vi "Format CSV.vi"(8 "error in (no error)":errorcluster, 9 "delimiter":string=",", 10 "CSV File Input":path, 11 "Original CSV Format":enum16{"Format A", "Format B"}(ring)) -> (0 "error out":errorcluster, 1 "Parcel Length":i32[](array[numeric]), 2 "All Terminal Data":T1(array[cluster]))   [LabVIEW 2017] (continued)
"44:49.4", "44:49.5", "44:49.5", "44:49.5", "44:49.6", "44:49.6", "44:49.6", "44:49.7", "44:49.7", "44:49.7", "44:49.8", "44:49.8", "44:49.8", "44:49.9", "44:49.9", "44:49.9", "44:50.0", "44:50.0", "44:50.0", "44:50.1", "44:50.1", "44:50.1", "44:50.2", "44:50.2", "44:50.2", "44:50.3", "44:50.3", "44:50.3", "44:50.4", "44:50.4", "44:50.4", "44:50.5", "44:50.5", "44:50.5", "44:50.6", "44:50.6", "44:50.6", "44:50.7", "44:50.7", "44:50.7", "44:50.8", "44:50.8", "44:50.8", "44:50.9", "44:50.9", "44:50.9", "44:51.0", "44:51.0", "44:51.0", "44:51.1", "44:51.1", "44:51.1", "44:51.2", "44:51.2", "44:51.2", "44:51.3", "44:51.3", "44:51.3", "44:51.4", "44:51.4", "44:51.4", "44:51.5", "44:51.5", "44:51.5", "44:51.6", "44:51.6", "44:51.6", "44:51.7", "44:51.7", "44:51.7", "44:51.8", "44:51.8", "44:51.8", "44:51.9", "44:51.9", "44:51.9", "44:52.0", "44:52.0", "44:52.0", "44:52.1", "44:52.1", "44:52.1", "44:52.2", "44:52.2", "44:52.2", "44:52.3", "44:52.3", "44:52.3", "44:52.4", "44:52.4", "44:52.4", "44:52.5", "44:52.5", "44:52.5", "44:52.6", "44:52.6", "44:52.6", "44:52.7", "44:52.7", "44:52.7", "44:52.8", "44:52.8", "44:52.8", "44:52.9", "44:52.9", "44:52.9", "44:53.0", "44:53.0", "44:53.0", "44:53.1", "44:53.1", "44:53.1", "44:53.2", "44:53.2", "44:53.2", "44:53.3", "44:53.3", "44:53.3", "44:53.4", "44:53.4", "44:53.4", "44:53.5", "44:53.5", "44:53.5", "44:53.6", "44:53.6", "44:53.6", "44:53.7", "44:53.7", "44:53.7", "44:53.8", "44:53.8", "44:53.8", "44:53.9", "44:53.9", "44:53.9", "44:54.0", "44:54.0", "44:54.0", "44:54.1", "44:54.1", "44:54.1", "44:54.2", "44:54.2", "44:54.2", "44:54.3", "44:54.3", "44:54.3", "44:54.4", "44:54.4", "44:54.4", "44:54.5", "44:54.5", "44:54.5", "44:54.6", "44:54.6", "44:54.6", "44:54.7", "44:54.7", "44:54.7", "44:54.8", "44:54.8", "44:54.8", "44:54.9", "44:54.9", "44:54.9", "44:55.0", "44:55.0", "44:55.0", "44:55.1", "44:55.1", "44:55.1", "44:55.2", "44:55.2", "44:55.2", "44:55.3", "44:55.3", "44:55.3", "44:55.4", "44:55.4", "44:55.4", "44:55.5", "44:55.5", "44:55.5", "44:55.6", "44:55.6", "44:55.6", "44:55.7", "44:55.7", "44:55.7", "44:55.8", "44:55.8", "44:55.8", "44:55.9", "44:55.9", "44:55.9", "44:56.0", "44:56.0", "44:56.0", "44:56.1", "44:56.1", "44:56.1", "44:56.2", "44:56.2", "44:56.2", "44:56.3", "44:56.3", "44:56.3", "44:56.4", "44:56.4", "44:56.4", "44:56.5", "44:56.5", "44:56.5", "44:56.6", "44:56.6", "44:56.6", "44:56.7", "44:56.7", "44:56.7", "44:56.8", "44:56.8", "44:56.8", "44:56.9", "44:56.9", "44:56.9", "44:57.0", "44:57.0", "44:57.0", "44:57.1", "44:57.1", "44:57.1", "44:57.2", "44:57.2", "44:57.2", "44:57.3", "44:57.3", "44:57.3", "44:57.4", "44:57.4", "44:57.4", "44:57.5", "44:57.5", "44:57.5", "44:57.6", "44:57.6", "44:57.6", "44:57.7", "44:57.7", "44:57.7", "44:57.8", "44:57.8", "44:57.8", "44:57.9", "44:57.9", "44:57.9", "44:58.0", "44:58.0", "44:58.0", "44:58.1", "44:58.1", "44:58.1", "44:58.2", "44:58.2", "44:58.2", "44:58.3", "44:58.3", "44:58.3", "44:58.4", "44:58.4", "44:58.4", "44:58.5", "44:58.5", "44:58.5", "44:58.6", "44:58.6", "44:58.6", "44:58.7", "44:58.7", "44:58.7", "44:58.8", "44:58.8", "44:58.8", "44:58.9", "44:58.9", "44:58.9", "44:59.0", "44:59.0", "44:59.0", "44:59.1", "44:59.1", "44:59.1", "44:59.2", "44:59.2", "44:59.2", "44:59.3", "44:59.3", "44:59.3", "44:59.4", "44:59.4", "44:59.4", "44:59.5", "44:59.5", "44:59.5", "44:59.6", "44:59.6", "44:59.6", "44:59.7", "44:59.7", "44:59.7", "44:59.8", "44:59.8", "44:59.8", "44:59.9", "44:59.9", "44:59.9", "45:00.0", "45:00.0", "45:00.0", "45:00.1", "45:00.1", "45:00.1", "45:00.2", "45:00.2", "45:00.2", "45:00.3", "45:00.3", "45:00.3", "45:00.4", "45:00.4", "45:00.4", "45:00.5", "45:00.5", "45:00.5", "45:00.6", "45:00.6", "45:00.6", "45:00.7", "45:00.7", "45:00.7", "45:00.8", "45:00.8", "45:00.8", "45:00.9", "45:00.9", "45:00.9", "45:01.0", "45:01.0", "45:01.0", "45:01.1", "45:01.1", "45:01.1", "45:01.2", "45:01.2", "45:01.2", "45:01.3", "45:01.3", "45:01.3", "45:01.4", "45:01.4", "45:01.4", "45:01.5", "45:01.5", "45:01.5", "45:01.6", "45:01.6", "45:01.6", "45:01.7", "45:01.7", "45:01.7", "45:01.8", "45:01.8", "45:01.8", "45:01.9", "45:01.9", "45:01.9", "45:02.0", "45:02.0", "45:02.0", "45:02.1", "45:02.1", "45:02.1", "45:02.2", "45:02.2", "45:02.2", "45:02.3", "45:02.3", "45:02.3", "45:02.4", "45:02.4", "45:02.4", "45:02.5", "45:02.5", "45:02.5", "45:02.6", "45:02.6", "45:02.6", "45:02.7", "45:02.7", "45:02.7", "45:02.8", "45:02.8", "45:02.8", "45:02.9", "45:02.9", "45:02.9", "45:03.0", "45:03.0", "45:03.0", "45:03.1", "45:03.1", "45:03.1", "45:03.2", "45:03.2", "45:03.2", "45:03.3", "45:03.3", "45:03.3", "45:03.4", "45:03.4", "45:03.4", "45:03.5", "45:03.5", "45:03.5", "45:03.6", "45:03.6", "45:03.6", "45:03.7", "45:03.7", "45:03.7", "45:03.8", "45:03.8", "45:03.8", "45:03.9", "45:03.9", "45:03.9", "45:04.0", "45:04.0", "45:04.0", "45:04.1", "45:04.1", "45:04.1", "45:04.2", "45:04.2", "45:04.2", "45:04.3", "45:04.3", "45:04.3", "45:04.4", "45:04.4", "45:04.4", "45:04.5", "45:04.5", "45:04.5", "45:04.6", "45:04.6", "45:04.6", "45:04.7", "45:04.7", "45:04.7", "45:04.8", "45:04.8", "45:04.8", "45:04.9", "45:04.9", "45:04.9", "45:05.0", "45:05.0", "45:05.0", "45:05.1", "45:05.1", "45:05.1", "45:05.2", "45:05.2", "45:05.2", "45:05.3", "45:05.3", "45:05.3", "45:05.4", "45:05.4", "45:05.4", "45:05.5", "45:05.5", "45:05.5", "45:05.6", "45:05.6", "45:05.6", "45:05.7", "45:05.7", "45:05.7", "45:05.8", "45:05.8", "45:05.8", "45:05.9", "45:05.9", "45:05.9", "45:06.0", "45:06.0", "45:06.0", "45:06.1", "45:06.1", "45:06.1", "45:06.2", "45:06.2", "45:06.2", "45:06.3", "45:06.3", "45:06.3", "45:06.4", "45:06.4", "45:06.4", "45:06.5", "45:06.5", "45:06.5", "45:06.6", "45:06.6", "45:06.6", "45:06.7", "45:06.7", "45:06.7", "45:06.8", "45:06.8", "45:06.8", "45:06.9", "45:06.9", "45:06.9", "45:07.0", "45:07.0", "45:07.0", "45:07.1", "45:07.1", "45:07.1", "45:07.2", "45:07.2", "45:07.2", "45:07.3", "45:07.3", "45:07.3", "45:07.4", "45:07.4", "45:07.4", "45:07.5", "45:07.5", "45:07.5", "45:07.6", "45:07.6", "45:07.6", "45:07.7", "45:07.7", "45:07.7", "45:07.8", "45:07.8", "45:07.8", "45:07.9", "45:07.9", "45:07.9", "45:08.0", "45:08.0", "45:08.0", "45:08.1", "45:08.1", "45:08.1", "45:08.2", "45:08.2", "45:08.2", "45:08.3", "45:08.3", "45:08.3", "45:08.4", "45:08.4", "45:08.4", "45:08.5", "45:08.5", "45:08.5", "45:08.6", "45:08.6", "45:08.6", "45:08.7", "45:08.7", "45:08.7", "45:08.8", "45:08.8", "45:08.8", "45:08.9", "45:08.9", "45:08.9", "45:09.0", "45:09.0", "45:09.0", "45:09.1", "45:09.1", "45:09.1", "45:09.2", "45:09.2", "45:09.2", "45:09.3", "45:09.3", "45:09.3", "45:09.4", "45:09.4", "45:09.4", "45:09.5", "45:09.5", "45:09.5", "45:09.6", "45:09.6", "45:09.6", "45:09.7", "45:09.7", "45:09.7", "45:09.8", "45:09.8", "45:09.8", "45:09.9", "45:09.9", "45:09.9", "45:10.0", "45:10.0", "45:10.0", "45:10.1", "45:10.1", "45:10.1", "45:10.2", "45:10.2", "45:10.2", "45:10.3", "45:10.3", "45:10.3", "45:10.4", "45:10.4", "45:10.4", "45:10.5", "45:10.5", "45:10.5", "45:10.6", "45:10.6", "45:10.6", "45:10.7", "45:10.7", "45:10.7", "45:10.8", "45:10.8", "45:10.8", "45:10.9", "45:10.9", "45:10.9", "45:11.0", "45:11.0", "45:11.0", "45:11.1", "45:11.1", "45:11.1", "45:11.2", "45:11.2", "45:11.2", "45:11.3", "45:11.3", "45:11.3", "45:11.4", "45:11.4", "45:11.4", "45:11.5", "45:11.5", "45:11.5", "45:11.6", "45:11.6", "45:11.6", "45:11.7", "45:11.7", "45:11.7", "45:11.8", "45:11.8", "45:11.8", "45:11.9", "45:11.9", "45:11.9", "45:12.0", "45:12.0", "45:12.0", "45:12.1", "45:12.1", "45:12.1", "45:12.2", "45:12.2", "45:12.2", "45:12.3", "45:12.3", "45:12.3", "45:12.4", "45:12.4", "45:12.4", "45:12.5", "45:12.5", "45:12.5", "45:12.6", "45:12.6", "45:12.6", "45:12.7", "45:12.7", "45:12.7", "45:12.8", "45:12.8", "45:12.8", "45:12.9", "45:12.9", "45:12.9", "45:13.0", "45:13.0", "45:13.0", "45:13.1", "45:13.1", "45:13.1", "45:13.2", "45:13.2", "45:13.2", "45:13.3", "45:13.3", "45:13.3", "45:13.4", "45:13.4", "45:13.4", "45:13.5", "45:13.5", "45:13.5", "45:13.6", "45:13.6", "45:13.6", "45:13.7", "45:13.7", "45:13.7", "45:13.8", "45:13.8", "45:13.8", "45:13.9", "45:13.9", "45:13.9", "45:14.0", "45:14.0", "45:14.0", "45:14.1", "45:14.1", "45:14.1", "45:14.2", "45:14.2", "45:14.2", "45:14.3", "45:14.3", "45:14.3", "45:14.4", "45:14.4", "45:14.4", "45:14.5", "45:14.5", "45:14.5", "45:14.6", "45:14.6", "45:14.6", "45:14.7", "45:14.7", "45:14.7", "45:14.8", "45:14.8", "45:14.8", "45:14.9", "45:14.9", "45:14.9", "45:15.0", "45:15.0", "45:15.0", "45:15.1", "45:15.1", "45:15.1", "45:15.2", "45:15.2", "45:15.2", "45:15.3", "45:15.3", "45:15.3", "45:15.4", "45:15.4", "45:15.4", "45:15.5", "45:15.5", "45:15.5", "45:15.6", "45:15.6", "45:15.6", "45:15.7", "45:15.7", "45:15.7", "45:15.8", "45:15.8", "45:15.8", "45:15.9", "45:15.9", "45:15.9", "45:16.0", "45:16.0", "45:16.0", "45:16.1", "45:16.1", "45:16.1", "45:16.2", "45:16.2", "45:16.2", "45:16.3", "45:16.3", "45:16.3", "45:16.4", "45:16.4", "45:16.4", "45:16.5", "45:16.5", "45:16.5", "45:16.6", "45:16.6", "45:16.6", "45:16.7", "45:16.7", "45:16.7", "45:16.8", "45:16.8", "45:16.8", "45:16.9", "45:16.9", "45:16.9", "45:17.0", "45:17.0", "45:17.0", "45:17.1", "45:17.1", "45:17.1", "45:17.2", "45:17.2", "45:17.2", "45:17.3", "45:17.3", "45:17.3", "45:17.4", "45:17.4", "45:17.4", "45:17.5", "45:17.5", "45:17.5", "45:17.6", "45:17.6", "45:17.6", "45:17.7", "45:17.7", "45:17.7", "45:17.8", "45:17.8", "45:17.8", "45:17.9", "45:17.9", "45:17.9", "45:18.0", "45:18.0", "45:18.0", "45:18.1", "45:18.1", "45:18.1", "45:18.2", "45:18.2", "45:18.2", "45:18.3", "45:18.3", "45:18.3", "45:18.4", "45:18.4", "45:18.4", "45:18.5", "45:18.5", "45:18.5", "45:18.6", "45:18.6", "45:18.6", "45:18.7", "45:18.7", "45:18.7", "45:18.8", "45:18.8", "45:18.8", "45:18.9", "45:18.9", "45:18.9", "45:19.0", "45:19.0", "45:19.0", "45:19.1", "45:19.1", "45:19.1", "45:19.2", "45:19.2", "45:19.2", "45:19.3", "45:19.3", "45:19.3", "45:19.4", "45:19.4", "45:19.4", "45:19.5", "45:19.5", "45:19.5", "45:19.6", "45:19.6", "45:19.6", "45:19.7", "45:19.7", "45:19.7", "45:19.8", "45:19.8", "45:19.8", "45:19.9", "45:19.9", "45:19.9", "45:20.0", "45:20.0", "45:20.0", "45:20.1", "45:20.1", "45:20.1", "45:20.2", "45:20.2", "45:20.2", "45:20.3", "45:20.3", "45:20.3", "45:20.4", "45:20.4", "45:20.4", "45:20.5", "45:20.5", "45:20.5", "45:20.6", "45:20.6", "45:20.6", "45:20.7", "45:20.7", "45:20.7", "45:20.8", "45:20.8", "45:20.8", "45:20.9", "45:20.9", "45:20.9", "45:21.0", "45:21.0", "45:21.0", "45:21.1", "45:21.1", "45:21.1", "45:21.2", "45:21.2", "45:21.2", "45:21.3", "45:21.3", "45:21.3", "45:21.4", "45:21.4", "45:21.4", "45:21.5", "45:21.5", "45:21.5", "45:21.6", "45:21.6", "45:21.6", "45:21.7", "45:21.7", "45:21.7", "45:21.8", "45:21.8", "45:21.8", "45:21.9", "45:21.9", "45:21.9", "45:22.0", "45:22.0", "45:22.0", "45:22.1", "45:22.1", "45:22.1", "45:22.2", "45:22.2", "45:22.2", "45:22.3", "45:22.3", "45:22.3", "45:22.4", "45:22.4", "45:22.4", "45:22.5", "45:22.5", "45:22.5", "45:22.6", "45:22.6", "45:22.6", "45:22.7", "45:22.7", "45:22.7", "45:22.8", "45:22.8", "45:22.8", "45:22.9", "45:22.9", "45:22.9", "45:23.0", "45:23.0", "45:23.0", "45:23.1", "45:23.1", "45:23.1", "45:23.2", "45:23.2", "45:23.2", "45:23.3", "45:23.3", "45:23.3", "45:23.4", "45:23.4", "45:23.4", "45:23.5", "45:23.5", "45:23.5", "45:23.6", "45:23.6", "45:23.6", "45:23.7", "45:23.7", "45:23.7", "45:23.8", "45:23.8", "45:23.8", "45:23.9", "45:23.9", "45:23.9", "45:24.0", "45:24.0", "45:24.0", "45:24.1", "45:24.1", "45:24.1", "45:24.2", "45:24.2", "45:24.2", "45:24.3", "45:24.3", "45:24.3", "45:24.4", "45:24.4", "45:24.4", "45:24.5", "45:24.5", "45:24.5", "45:24.6", "45:24.6", "45:24.6", "45:24.7", "45:24.7", "45:24.7", "45:24.8", "45:24.8", "45:24.8", "45:24.9", "45:24.9", "45:24.9", "45:25.0", "45:25.0", "45:25.0", "45:25.1", "45:25.1", "45:25.1", "45:25.2", "45:25.2", "45:25.2", "45:25.3", "45:25.3", "45:25.3", "45:25.4", "45:25.4", "45:25.4", "45:25.5", "45:25.5", "45:25.5", "45:25.6", "45:25.6", "45:25.6", "45:25.7", "45:25.7", "45:25.7", "45:25.8", "45:25.8", "45:25.8", "45:25.9", "45:25.9", "45:25.9", "45:26.0", "45:26.0", "45:26.0", "45:26.1", "45:26.1", "45:26.1", "45:26.2", "45:26.2", "45:26.2", "45:26.3", "45:26.3", "45:26.3", "45:26.4", "45:26.4", "45:26.4", "45:26.5", "45:26.5", "45:26.5", "45:26.6", "45:26.6", "45:26.6", "45:26.7", "45:26.7", "45:26.7", "45:26.8", "45:26.8", "45:26.8", "45:26.9", "45:26.9", "45:26.9", "45:27.0", "45:27.0", "45:27.0", "45:27.1", "45:27.1", "45:27.1", "45:27.2", "45:27.2", "45:27.2", "45:27.3", "45:27.3", "45:27.3", "45:27.4", "45:27.4", "45:27.4", "45:27.5", "45:27.5", "45:27.5", "45:27.6", "45:27.6", "45:27.6", "45:27.7", "45:27.7", "45:27.7", "45:27.8", "45:27.8", "45:27.8", "45:27.9", "45:27.9", "45:27.9", "45:28.0", "45:28.0", "45:28.0", "45:28.1", "45:28.1", "45:28.1", "45:28.2", "45:28.2", "45:28.2", "45:28.3", "45:28.3", "45:28.3", "45:28.4", "45:28.4", "45:28.4", "45:28.5", "45:28.5", "45:28.5", "45:28.6", "45:28.6", "45:28.6", "45:28.7", "45:28.7", "45:28.7", "45:28.8", "45:28.8", "45:28.8", "45:28.9", "45:28.9", "45:28.9", "45:29.0", "45:29.0", "45:29.0", "45:29.1", "45:29.1", "45:29.1", "45:29.2", "45:29.2", "45:29.2", "45:29.3", "45:29.3", "45:29.3", "45:29.4", "45:29.4", "45:29.4", "45:29.5", "45:29.5", "45:29.5", "45:29.6", "45:29.6", "45:29.6", "45:29.7", "45:29.7", "45:29.7", "45:29.8", "45:29.8", "45:29.8", "45:29.9", "45:29.9", "45:29.9", "45:30.0", "45:30.0", "45:30.0", "45:30.1", "45:30.1", "45:30.1", "45:30.2", "45:30.2", "45:30.2", "45:30.3", "45:30.3", "45:30.3", "45:30.4", "45:30.4", "45:30.4", "45:30.5", "45:30.5", "45:30.5", "45:30.6", "45:30.6", "45:30.6", "45:30.7", "45:30.7", "45:30.7", "45:30.8", "45:30.8", "45:30.8", "45:30.9", "45:30.9", "45:30.9", "45:31.0", "45:31.0", "45:31.0", "45:31.1", "45:31.1", "45:31.1", "45:31.2", "45:31.2", "45:31.2", "45:31.3", "45:31.3", "45:31.3", "45:31.4", "45:31.4", "45:31.4", "45:31.5", "45:31.5", "45:31.5", "45:31.6", "45:31.6", "45:31.6", "45:31.7", "45:31.7", "45:31.7", "45:31.8", "45:31.8", "45:31.8", "45:31.9", "45:31.9", "45:31.9", "45:32.0", "45:32.0", "45:32.0", "45:32.1", "45:32.1", "45:32.1", "45:32.2", "45:32.2", "45:32.2", "45:32.3", "45:32.3", "45:32.3", "45:32.4", "45:32.4", "45:32.4", "45:32.5", "45:32.5", "45:32.5", "45:32.6", "45:32.6", "45:32.6", "45:32.7", "45:32.7", "45:32.7", "45:32.8", "45:32.8", "45:32.8", "45:32.9", "45:32.9", "45:32.9", "45:33.0", "45:33.0", "45:33.0", "45:33.1", "45:33.1", "45:33.1", "45:33.2", "45:33.2", "45:33.2", "45:33.3", "45:33.3", "45:33.3", "45:33.4", "45:33.4", "45:33.4", "45:33.5", "45:33.5", "45:33.5", "45:33.6", "45:33.6", "45:33.6", "45:33.7", "45:33.7", "45:33.7", "45:33.8", "45:33.8", "45:33.8", "45:33.9", "45:33.9", "45:33.9", "45:34.0", "45:34.0", "45:34.0", "45:34.1", "45:34.1", "45:34.1", "45:34.2", "45:34.2", "45:34.2", "45:34.3", "45:34.3", "45:34.3", "45:34.4", "45:34.4", "45:34.4", "45:34.5", "45:34.5", "45:34.5", "45:34.6", "45:34.6", "45:34.6", "45:34.7", "45:34.7", "45:34.7", "45:34.8", "45:34.8", "45:34.8", "45:34.9", "45:34.9", "45:34.9", "45:35.0", "45:35.0", "45:35.0", "45:35.1", "45:35.1", "45:35.1", "45:35.2", "45:35.2", "45:35.2", "45:35.3", "45:35.3", "45:35.3", "45:35.4", "45:35.4", "45:35.4", "45:35.5", "45:35.5", "45:35.5", "45:35.6", "45:35.6", "45:35.6", "45:35.7", "45:35.7", "45:35.7", "45:35.8", "45:35.8", "45:35.8", "45:35.9", "45:35.9", "45:35.9", "45:36.0", "45:36.0", "45:36.0", "45:36.1", "45:36.1", "45:36.1", "45:36.2", "45:36.2", "45:36.2", "45:36.3", "45:36.3", "45:36.3", "45:36.4", "45:36.4", "45:36.4", "45:36.5", "45:36.5", "45:36.5", "45:36.6", "45:36.6", "45:36.6", "45:36.7", "45:36.7", "45:36.7", "45:36.8", "45:36.8", "45:36.8", "45:36.9", "45:36.9", "45:36.9", "45:37.0", "45:37.0", "45:37.0", "45:37.1", "45:37.1", "45:37.1", "45:37.2", "45:37.2", "45:37.2", "45:37.3", "45:37.3", "45:37.3", "45:37.4", "45:37.4", "45:37.4", "45:37.5", "45:37.5", "45:37.5", "45:37.6", "45:37.6", "45:37.6", "45:37.7", "45:37.7", "45:37.7", "45:37.8", "45:37.8", "45:37.8", "45:37.9", "45:37.9", "45:37.9", "45:38.0", "45:38.0", "45:38.0", "45:38.1", "45:38.1", "45:38.1", "45:38.2", "45:38.2", "45:38.2", "45:38.3", "45:38.3", "45:38.3", "45:38.4", "45:38.4", "45:38.4", "45:38.5", "45:38.5", "45:38.5", "45:38.6", "45:38.6", "45:38.6", "45:38.7", "45:38.7", "45:38.7", "45:38.8", "45:38.8", "45:38.8", "45:38.9", "45:38.9", "45:38.9", "45:39.0", "45:39.0", "45:39.0", "45:39.1", "45:39.1", "45:39.1", "45:39.2", "45:39.2", "45:39.2", "45:39.3", "45:39.3", "45:39.3", "45:39.4", "45:39.4", "45:39.4", "45:39.5", "45:39.5", "45:39.5", "45:39.6", "45:39.6", "45:39.6", "45:39.7", "45:39.7", "45:39.7", "45:39.8", "45:39.8", "45:39.8", "45:39.9", "45:39.9", "45:39.9", "45:40.0", "45:40.0", "45:40.0", "45:40.1", "45:40.1", "45:40.1", "45:40.2", "45:40.2", "45:40.2", "45:40.3", "45:40.3", "45:40.3", "45:40.4", "45:40.4", "45:40.4", "45:40.5", "45:40.5", "45:40.5", "45:40.6", "45:40.6", "45:40.6", "45:40.7", "45:40.7", "45:40.7", "45:40.8", "45:40.8", "45:40.8", "45:40.9", "45:40.9", "45:40.9", "45:41.0", "45:41.0", "45:41.0", "45:41.1", "45:41.1", "45:41.1", "45:41.2", "45:41.2", "45:41.2", "45:41.3", "45:41.3", "45:41.3", "45:41.4", "45:41.4", "45:41.4", "45:41.5", "45:41.5", "45:41.5", "45:41.6", "45:41.6", "45:41.6", "45:41.7", "45:41.7", "45:41.7", "45:41.8", "45:41.8", "45:41.8", "45:41.9", "45:41.9", "45:41.9", "45:42.0", "45:42.0", "45:42.0", "45:42.1", "45:42.1", "45:42.1", "45:42.2", "45:42.2", "45:42.2", "45:42.3", "45:42.3", "45:42.3", "45:42.4", "45:42.4", "45:42.4", "45:42.5", "45:42.5", "45:42.5", "45:42.6", "45:42.6", "45:42.6", "45:42.7", "45:42.7", "45:42.7", "45:42.8", "45:42.8", "45:42.8", "45:42.9", "45:42.9", "45:42.9", "45:43.0", "45:43.0", "45:43.0", "45:43.1", "45:43.1", "45:43.1", "45:43.2", "45:43.2", "45:43.2", "45:43.3", "45:43.3", "45:43.3", "45:43.4", "45:43.4", "45:43.4", "45:43.5", "45:43.5", "45:43.5", "45:43.6", "45:43.6", "45:43.6", "45:43.7", "45:43.7", "45:43.7", "45:43.8", "45:43.8", "45:43.8", "45:43.9", "45:43.9", "45:43.9", "45:44.0", "45:44.0", "45:44.0", "45:44.1", "45:44.1", "45:44.1", "45:44.2", "45:44.2", "45:44.2", "45:44.3", "45:44.3", "45:44.3", "45:44.4", "45:44.4", "45:44.4", "45:44.5", "45:44.5", "45:44.5", "45:44.6", "45:44.6", "45:44.6", "45:44.7", "45:44.7", "45:44.7", "45:44.8", "45:44.8", "45:44.8", "45:44.9", "45:44.9", "45:44.9", "45:45.0", "45:45.0", "45:45.0", "45:45.1", "45:45.1", "45:45.1", "45:45.2", "45:45.2", "45:45.2", "45:45.3", "45:45.3", "45:45.3", "45:45.4", "45:45.4", "45:45.4", "45:45.5", "45:45.5", "45:45.5", "45:45.6", "45:45.6", "45:45.6", "45:45.7", "45:45.7", "45:45.7", "45:45.8", "45:45.8", "45:45.8", "45:45.9", "45:45.9", "45:45.9", "45:46.0", "45:46.0", "45:46.0", "45:46.1", "45:46.1", "45:46.1", "45:46.2", "45:46.2", "45:46.2", "45:46.3", "45:46.3", "45:46.3", "45:46.4", "45:46.4", "45:46.4", "45:46.5", "45:46.5", "45:46.5", "45:46.6", "45:46.6", "45:46.6", "45:46.7", "45:46.7", "45:46.7", "45:46.8", "45:46.8", "45:46.8", "45:46.9", "45:46.9", "45:46.9", "45:47.0", "45:47.0", "45:47.0", "45:47.1", "45:47.1", "45:47.1", "45:47.2", "45:47.2", "45:47.2", "45:47.3", "45:47.3", "45:47.3", "45:47.4", "45:47.4", "45:47.4", "45:47.5", "45:47.5", "45:47.5", "45:47.6", "45:47.6", "45:47.6", "45:47.7", "45:47.7", "45:47.7", "45:47.8", "45:47.8", "45:47.8", "45:47.9", "45:47.9", "45:47.9", "45:48.0", "45:48.0", "45:48.0", "45:48.1", "45:48.1", "45:48.1", "45:48.2", "45:48.2", "45:48.2", "45:48.3", "45:48.3", "45:48.3", "45:48.4", "45:48.4", "45:48.4", "45:48.5", "45:48.5", "45:48.5", "45:48.6", "45:48.6", "45:48.6", "45:48.7", "45:48.7", "45:48.7", "45:48.8", "45:48.8", "45:48.8", "45:48.9", "45:48.9", "45:48.9", "45:49.0", "45:49.0", "45:49.0", "45:49.1", "45:49.1", "45:49.1", "45:49.2", "45:49.2", "45:49.2", "45:49.3", "45:49.3", "45:49.3", "45:49.4", "45:49.4", "45:49.4", "45:49.5", "45:49.5", "45:49.5", "45:49.6", "45:49.6", "45:49.6", "45:49.7", "45:49.7", "45:49.7", "45:49.8", "45:49.8", "45:49.8", "45:49.9", "45:49.9", "45:49.9", "45:50.0", "45:50.0", "45:50.0", "45:50.1", "45:50.1", "45:50.1", "45:50.2", "45:50.2", "45:50.2", "45:50.3", "45:50.3", "45:50.3", "45:50.4", "45:50.4", "45:50.4", "45:50.5", "45:50.5", "45:50.5", "45:50.6", "45:50.6", "45:50.6", "45:50.7", "45:50.7", "45:50.7", "45:50.8", "45:50.8", "45:50.8", "45:50.9", "45:50.9", "45:50.9", "45:51.0", "45:51.0", "45:51.0", "45:51.1", "45:51.1", "45:51.1", "45:51.2", "45:51.2", "45:51.2", "45:51.3", "45:51.3", "45:51.3", "45:51.4", "45:51.4", "45:51.4", "45:51.5", "45:51.5", "45:51.5", "45:51.6", "45:51.6", "45:51.6", "45:51.7", "45:51.7", "45:51.7", "45:51.8", "45:51.8", "45:51.8", "45:51.9", "45:51.9", "45:51.9", "45:52.0", "45:52.0", "45:52.0", "45:52.1", "45:52.1", "45:52.1", "45:52.2", "45:52.2", "45:52.2", "45:52.3", "45:52.3", "45:52.3", "45:52.4", "45:52.4", "45:52.4", "45:52.5", "45:52.5", "45:52.5", "45:52.6", "45:52.6", "45:52.6", "45:52.7", "45:52.7", "45:52.7", "45:52.8", "45:52.8", "45:52.8", "45:52.9", "45:52.9", "45:52.9", "45:53.0", "45:53.0", "45:53.0", "45:53.1", "45:53.1", "45:53.1", "45:53.2", "45:53.2", "45:53.2", "45:53.3", "45:53.3", "45:53.3", "45:53.4", "45:53.4", "45:53.4", "45:53.5", "45:53.5", "45:53.5", "45:53.6", "45:53.6", "45:53.6", "45:53.7", "45:53.7", "45:53.7", "45:53.8", "45:53.8", "45:53.8", "45:53.9", "45:53.9", "45:53.9", "45:54.0", "45:54.0", "45:54.0", "45:54.1", "45:54.1", "45:54.1", "45:54.2", "45:54.2", "45:54.2", "45:54.3", "45:54.3", "45:54.3", "45:54.4", "45:54.4", "45:54.4", "45:54.5", "45:54.5", "45:54.5", "45:54.6", "45:54.6", "45:54.6", "45:54.7", "45:54.7", "45:54.7", "45:54.8", "45:54.8", "45:54.8", "45:54.9", "45:54.9", "45:54.9", "45:55.0", "45:55.0", "45:55.0", "45:55.1", "45:55.1", "45:55.1", "45:55.2", "45:55.2", "45:55.2", "45:55.3", "45:55.3", "45:55.3", "45:55.4", "45:55.4", "45:55.4", "45:55.5", "45:55.5", "45:55.5", "45:55.6", "45:55.6", "45:55.6", "45:55.7", "45:55.7", "45:55.7", "45:55.8", "45:55.8", "45:55.8", "45:55.9", "45:55.9", "45:55.9", "45:56.0", "45:56.0", "45:56.0", "45:56.1", "45:56.1", "45:56.1", "45:56.2", "45:56.2", "45:56.2", "45:56.3", "45:56.3", "45:56.3", "45:56.4", "45:56.4", "45:56.4", "45:56.5", "45:56.5", "45:56.5", "45:56.6", "45:56.6", "45:56.6", "45:56.7", "45:56.7", "45:56.7", "45:56.8", "45:56.8", "45:56.8", "45:56.9", "45:56.9", "45:56.9", "45:57.0", "45:57.0", "45:57.0", "45:57.1", "45:57.1", "45:57.1", "45:57.2", "45:57.2", "45:57.2", "45:57.3", "45:57.3", "45:57.3", "45:57.4", "45:57.4", "45:57.4", "45:57.5", "45:57.5", "45:57.5", "45:57.6", "45:57.6", "45:57.6", "45:57.7", "45:57.7", "45:57.7", "45:57.8", "45:57.8", "45:57.8", "45:57.9", "45:57.9", "45:57.9", "45:58.0", "45:58.0", "45:58.0", "45:58.1", "45:58.1", "45:58.1", "45:58.2", "45:58.2", "45:58.2", "45:58.3", "45:58.3", "45:58.3", "45:58.4", "45:58.4", "45:58.4", "45:58.5", "45:58.5", "45:58.5", "45:58.6", "45:58.6", "45:58.6", "45:58.7", "45:58.7", "45:58.7", "45:58.8", "45:58.8", "45:58.8", "45:58.9", "45:58.9", "45:58.9", "45:59.0", "45:59.0", "45:59.0", "45:59.1", "45:59.1", "45:59.1", "45:59.2", "45:59.2", "45:59.2", "45:59.3", "45:59.3", "45:59.3", "45:59.4", "45:59.4", "45:59.4", "45:59.5", "45:59.5", "45:59.5", "45:59.6", "45:59.6", "45:59.6", "45:59.7", "45:59.7", "45:59.7", "45:59.8", "45:59.8", "45:59.8", "45:59.9", "45:59.9", "45:59.9", "46:00.0", "46:00.0", "46:00.0", "46:00.1", "46:00.1", "46:00.1", "46:00.2", "46:00.2", "46:00.2", "46:00.3", "46:00.3", "46:00.3", "46:00.4", "46:00.4", "46:00.4", "46:00.5", "46:00.5", "46:00.5", "46:00.6", "46:00.6", "46:00.6", "46:00.7", "46:00.7", "46:00.7", "46:00.8", "46:00.8", "46:00.8", "46:00.9", "46:00.9", "46:00.9", "46:01.0", "46:01.0", "46:01.0", "46:01.1", "46:01.1", "46:01.1", "46:01.2", "46:01.2", "46:01.2", "46:01.3", "46:01.3", "46:01.3", "46:01.4", "46:01.4", "46:01.4", "46:01.5", "46:01.5", "46:01.5", "46:01.6", "46:01.6", "46:01.6", "46:01.7", "46:01.7", "46:01.7", "46:01.8", "46:01.8", "46:01.8", "46:01.9", "46:01.9", "46:01.9", "46:02.0", "46:02.0", "46:02.0", "46:02.1", "46:02.1", "46:02.1", "46:02.2", "46:02.2", "46:02.2", "46:02.3", "46:02.3", "46:02.3", "46:02.4", "46:02.4", "46:02.4", "46:02.5", "46:02.5", "46:02.5", "46:02.6", "46:02.6", "46:02.6", "46:02.7", "46:02.7", "46:02.7", "46:02.8", "46:02.8", "46:02.8", "46:02.9", "46:02.9", "46:02.9", "46:03.0", "46:03.0", "46:03.0", "46:03.1", "46:03.1", "46:03.1", "46:03.2", "46:03.2", "46:03.2", "46:03.3", "46:03.3", "46:03.3", "46:03.4", "46:03.4", "46:03.4", "46:03.5", "46:03.5", "46:03.5", "46:03.6", "46:03.6", "46:03.6", "46:03.7", "46:03.7", "46:03.7", "46:03.8", "46:03.8", "46:03.8", "46:03.9", "46:03.9", "46:03.9", "46:04.0", "46:04.0", "46:04.0", "46:04.1", "46:04.1", "46:04.1", "46:04.2", "46:04.2", "46:04.2", "46:04.3", "46:04.3", "46:04.3", "46:04.4", "46:04.4", "46:04.4", "46:04.5", "46:04.5", "46:04.5", "46:04.6", "46:04.6", "46:04.6", "46:04.7", "46:04.7", "46:04.7", "46:04.8", "46:04.8", "46:04.8", "46:04.9", "46:04.9", "46:04.9", "46:05.0", "46:05.0", "46:05.0", "46:05.1", "46:05.1", "46:05.1", "46:05.2", "46:05.2", "46:05.2", "46:05.3", "46:05.3", "46:05.3", "46:05.4", "46:05.4", "46:05.4", "46:05.5", "46:05.5", "46:05.5", "46:05.6", "46:05.6", "46:05.6", "46:05.7", "46:05.7", "46:05.7", "46:05.8", "46:05.8", "46:05.8", "46:05.9", "46:05.9", "46:05.9", "46:06.0", "46:06.0", "46:06.0", "46:06.1", "46:06.1", "46:06.1", "46:06.2", "46:06.2", "46:06.2", "46:06.3", "46:06.3", "46:06.3", "46:06.4", "46:06.4", "46:06.4", "46:06.5", "46:06.5", "46:06.5", "46:06.6", "46:06.6", "46:06.6", "46:06.7", "46:06.7", "46:06.7", "46:06.8", "46:06.8", "46:06.8", "46:06.9", "46:06.9", "46:06.9", "46:07.0", "46:07.0", "46:07.0", "46:07.1", "46:07.1", "46:07.1", "46:07.2", "46:07.2", "46:07.2", "46:07.3", "46:07.3", "46:07.3", "46:07.4", "46:07.4", "46:07.4", "46:07.5", "46:07.5", "46:07.5", "46:07.6", "46:07.6", "46:07.6", "46:07.7", "46:07.7", "46:07.7", "46:07.8", "46:07.8", "46:07.8", "46:07.9", "46:07.9", "46:07.9", "46:08.0", "46:08.0", "46:08.0", "46:08.1", "46:08.1", "46:08.1", "46:08.2", "46:08.2", "46:08.2", "46:08.3", "46:08.3", "46:08.3", "46:08.4", "46:08.4", "46:08.4", "46:08.5", "46:08.5", "46:08.5", "46:08.6", "46:08.6", "46:08.6", "46:08.7", "46:08.7", "46:08.7", "46:08.8", "46:08.8", "46:08.8", "46:08.9", "46:08.9", "46:08.9", "46:09.0", "46:09.0", "46:09.0", "46:09.1", "46:09.1", "46:09.1", "46:09.2", "46:09.2", "46:09.2", "46:09.3", "46:09.3", "46:09.3", "46:09.4", "46:09.4", "46:09.4", "46:09.5", "46:09.5", "46:09.5", "46:09.6", "46:09.6", "46:09.6", "46:09.7", "46:09.7", "46:09.7", "46:09.8", "46:09.8", "46:09.8", "46:09.9", "46:09.9", "46:09.9", "46:10.0", "46:10.0", "46:10.0", "46:10.1", "46:10.1", "46:10.1", "46:10.2", "46:10.2", "46:10.2", "46:10.3", "46:10.3", "46:10.3", "46:10.4", "46:10.4", "46:10.4", "46:10.5", "46:10.5", "46:10.5", "46:10.6", "46:10.6", "46:10.6", "46:10.7", "46:10.7", "46:10.7", "46:10.8", "46:10.8", "46:10.8", "46:10.9", "46:10.9", "46:10.9", "46:11.0", "46:11.0", "46:11.0", "46:11.1", "46:11.1", "46:11.1", "46:11.2", "46:11.2", "46:11.2", "46:11.3", "46:11.3", "46:11.3", "46:11.4", "46:11.4", "46:11.4", "46:11.5", "46:11.5", "46:11.5", "46:11.6", "46:11.6", "46:11.6", "46:11.7", "46:11.7", "46:11.7", "46:11.8", "46:11.8", "46:11.8", "46:11.9", "46:11.9", "46:11.9", "46:12.0", "46:12.0", "46:12.0", "46:12.1", "46:12.1", "46:12.1", "46:12.2", "46:12.2", "46:12.2", "46:12.3", "46:12.3", "46:12.3", "46:12.4", "46:12.4", "46:12.4", "46:12.5", "46:12.5", "46:12.5", "46:12.6", "46:12.6", "46:12.6", "46:12.7", "46:12.7", "46:12.7", "46:12.8", "46:12.8", "46:12.8", "46:12.9", "46:12.9", "46:12.9", "46:13.0", "46:13.0", "46:13.0", "46:13.1", "46:13.1", "46:13.1", "46:13.2", "46:13.2", "46:13.2", "46:13.3", "46:13.3", "46:13.3", "46:13.4", "46:13.4", "46:13.4", "46:13.5", "46:13.5", "46:13.5", "46:13.6", "46:13.6", "46:13.6", "46:13.7", "46:13.7", "46:13.7", "46:13.8", "46:13.8", "46:13.8", "46:13.9", "46:13.9", "46:13.9", "46:14.0", "46:14.0", "46:14.0", "46:14.1", "46:14.1", "46:14.1", "46:14.2", "46:14.2", "46:14.2", "46:14.3", "46:14.3", "46:14.3", "46:14.4", "46:14.4", "46:14.4", "46:14.5", "46:14.5", "46:14.5", "46:14.6", "46:14.6", "46:14.6", "46:14.7", "46:14.7", "46:14.7", "46:14.8", "46:14.8", "46:14.8", "46:14.9", "46:14.9", "46:14.9", "46:15.0", "46:15.0", "46:15.0", "46:15.1", "46:15.1", "46:15.1", "46:15.2", "46:15.2", "46:15.2", "46:15.3", "46:15.3", "46:15.3", "46:15.4", "46:15.4", "46:15.4", "46:15.5", "46:15.5", "46:15.5", "46:15.6", "46:15.6", "46:15.6", "46:15.7", "46:15.7", "46:15.7", "46:15.8", "46:15.8", "46:15.8", "46:15.9", "46:15.9", "46:15.9", "46:16.0", "46:16.0", "46:16.0", "46:16.1", "46:16.1", "46:16.1", "46:16.2", "46:16.2", "46:16.2", "46:16.3", "46:16.3", "46:16.3", "46:16.4", "46:16.4", "46:16.4", "46:16.5", "46:16.5", "46:16.5", "46:16.6", "46:16.6", "46:16.6", "46:16.7", "46:16.7", "46:16.7", "46:16.8", "46:16.8", "46:16.8", "46:16.9", "46:16.9", "46:16.9", "46:17.0", "46:17.0", "46:17.0", "46:17.1", "46:17.1", "46:17.1", "46:17.2", "46:17.2", "46:17.2", "46:17.3", "46:17.3", "46:17.3", "46:17.4", "46:17.4", "46:17.4", "46:17.5", "46:17.5", "46:17.5", "46:17.6", "46:17.6", "46:17.6", "46:17.7", "46:17.7", "46:17.7", "46:17.8", "46:17.8", "46:17.8", "46:17.9", "46:17.9", "46:17.9", "46:18.0", "46:18.0", "46:18.0", "46:18.1", "46:18.1", "46:18.1", "46:18.2", "46:18.2", "46:18.2", "46:18.3", "46:18.3", "46:18.3", "46:18.4", "46:18.4", "46:18.4", "46:18.5", "46:18.5", "46:18.5", "46:18.6", "46:18.6", "46:18.6", "46:18.7", "46:18.7", "46:18.7", "46:18.8", "46:18.8", "46:18.8", "46:18.9", "46:18.9", "46:18.9", "46:19.0", "46:19.0", "46:19.0", "46:19.1", "46:19.1", "46:19.1", "46:19.2", "46:19.2", "46:19.2", "46:19.3", "46:19.3", "46:19.3", "46:19.4", "46:19.4", "46:19.4", "46:19.5", "46:19.5", "46:19.5", "46:19.6", "46:19.6", "46:19.6", "46:19.7", "46:19.7", "46:19.7", "46:19.8", "46:19.8", "46:19.8", "46:19.9", "46:19.9", "46:19.9", "46:20.0", "46:20.0", "46:20.0", "46:20.1", "46:20.1", "46:20.1", "46:20.2", "46:20.2", "46:20.2", "46:20.3", "46:20.3", "46:20.3", "46:20.4", "46:20.4", "46:20.4", "46:20.5", "46:20.5", "46:20.5", "46:20.6", "46:20.6", "46:20.6", "46:20.7", "46:20.7", "46:20.7", "46:20.8", "46:20.8", "46:20.8", "46:20.9", "46:20.9", "46:20.9", "46:21.0", "46:21.0", "46:21.0", "46:21.1", "46:21.1", "46:21.1", "46:21.2", "46:21.2", "46:21.2", "46:21.3", "46:21.3", "46:21.3", "46:21.4", "46:21.4", "46:21.4", "46:21.5", "46:21.5", "46:21.5", "46:21.6", "46:21.6", "46:21.6", "46:21.7", "46:21.7", "46:21.7", "46:21.8", "46:21.8", "46:21.8", "46:21.9", "46:21.9", "46:21.9", "46:22.0", "46:22.0", "46:22.0", "46:22.1", "46:22.1", "46:22.1", "46:22.2", "46:22.2", "46:22.2", "46:22.3", "46:22.3", "46:22.3", "46:22.4", "46:22.4", "46:22.4", "46:22.5", "46:22.5", "46:22.5", "46:22.6", "46:22.6", "46:22.6", "46:22.7", "46:22.7", "46:22.7", "46:22.8", "46:22.8", "46:22.8", "46:22.9", "46:22.9", "46:22.9", "46:23.0", "46:23.0", "46:23.0", "46:23.1", "46:23.1", "46:23.1", "46:23.2", "46:23.2", "46:23.2", "46:23.3", "46:23.3", "46:23.3", "46:23.4", "46:23.4", "46:23.4", "46:23.5", "46:23.5", "46:23.5", "46:23.6", "46:23.6", "46:23.6", "46:23.7", "46:23.7", "46:23.7", "46:23.8", "46:23.8", "46:23.8", "46:23.9", "46:23.9", "46:23.9", "46:24.0", "46:24.0", "46:24.0", "46:24.1", "46:24.1", "46:24.1", "46:24.2", "46:24.2", "46:24.2", "46:24.3", "46:24.3", "46:24.3", "46:24.4", "46:24.4", "46:24.4", "46:24.5", "46:24.5", "46:24.5", "46:24.6", "46:24.6", "46:24.6", "46:24.7", "46:24.7", "46:24.7", "46:24.8", "46:24.8", "46:24.8", "46:24.9", "46:24.9", "46:24.9", "46:25.0", "46:25.0", "46:25.0", "46:25.1", "46:25.1", "46:25.1", "46:25.2", "46:25.2", "46:25.2", "46:25.3", "46:25.3", "46:25.3", "46:25.4", "46:25.4", "46:25.4", "46:25.5", "46:25.5", "46:25.5", "46:25.6", "46:25.6", "46:25.6", "46:25.7", "46:25.7", "46:25.7", "46:25.8", "46:25.8", "46:25.8", "46:25.9", "46:25.9", "46:25.9", "46:26.0", "46:26.0", "46:26.0", "46:26.1", "46:26.1", "46:26.1", "46:26.2", "46:26.2", "46:26.2", "46:26.3", "46:26.3", "46:26.3", "46:26.4", "46:26.4", "46:26.4", "46:26.5", "46:26.5", "46:26.5", "46:26.6", "46:26.6", "46:26.6", "46:26.7", "46:26.7", "46:26.7", "46:26.8", "46:26.8", "46:26.8", "46:26.9", "46:26.9", "46:26.9", "46:27.0", "46:27.0", "46:27.0", "46:27.1", "46:27.1", "46:27.1", "46:27.2", "46:27.2", "46:27.2", "46:27.3", "46:27.3", "46:27.3", "46:27.4", "46:27.4", "46:27.4", "46:27.5", "46:27.5", "46:27.5", "46:27.6", "46:27.6", "46:27.6", "46:27.7", "46:27.7", "46:27.7", "46:27.8", "46:27.8", "46:27.8", "46:27.9", "46:27.9", "46:27.9", "46:28.0", "46:28.0", "46:28.0", "46:28.1", "46:28.1", "46:28.1", "46:28.2", "46:28.2", "46:28.2", "46:28.3", "46:28.3", "46:28.3", "46:28.4", "46:28.4", "46:28.4", "46:28.5", "46:28.5", "46:28.5", "46:28.6", "46:28.6", "46:28.6", "46:28.7", "46:28.7", "46:28.7", "46:28.8", "46:28.8", "46:28.8", "46:28.9", "46:28.9", "46:28.9", "46:29.0", "46:29.0", "46:29.0", "46:29.1", "46:29.1", "46:29.1", "46:29.2", "46:29.2", "46:29.2", "46:29.3", "46:29.3", "46:29.3", "46:29.4", "46:29.4", "46:29.4", "46:29.5", "46:29.5", "46:29.5", "46:29.6", "46:29.6", "46:29.6", "46:29.7", "46:29.7", "46:29.7", "46:29.8", "46:29.8", "46:29.8", "46:29.9", "46:29.9", "46:29.9", "46:30.0", "46:30.0", "46:30.0", "46:30.1", "46:30.1", "46:30.1", "46:30.2", "46:30.2", "46:30.2", "46:30.3", "46:30.3", "46:30.3", "46:30.4", "46:30.4", "46:30.4", "46:30.5", "46:30.5", "46:30.5", "46:30.6", "46:30.6", "46:30.6", "46:30.7", "46:30.7", "46:30.7", "46:30.8", "46:30.8", "46:30.8", "46:30.9", "46:30.9", "46:30.9", "46:31.0", "46:31.0", "46:31.0", "46:31.1", "46:31.1", "46:31.1", "46:31.2", "46:31.2", "46:31.2", "46:31.3", "46:31.3", "46:31.3", "46:31.4", "46:31.4", "46:31.4", "46:31.5", "46:31.5", "46:31.5", "46:31.6", "46:31.6", "46:31.6", "46:31.7", "46:31.7", "46:31.7", "46:31.8", "46:31.8", "46:31.8", "46:31.9", "46:31.9", "46:31.9", "46:32.0", "46:32.0", "46:32.0", "46:32.1", "46:32.1", "46:32.1", "46:32.2", "46:32.2", "46:32.2", "46:32.3", "46:32.3", "46:32.3", "46:32.4", "46:32.4", "46:32.4", "46:32.5", "46:32.5", "46:32.5", "46:32.6", "46:32.6", "46:32.6", "46:32.7", "46:32.7", "46:32.7", "46:32.8", "46:32.8", "46:32.8", "46:32.9", "46:32.9", "46:32.9", "46:33.0", "46:33.0", "46:33.0", "46:33.1", "46:33.1", "46:33.1", "46:33.2", "46:33.2", "46:33.2", "46:33.3", "46:33.3", "46:33.3", "46:33.4", "46:33.4", "46:33.4", "46:33.5", "46:33.5", "46:33.5", "46:33.6", "46:33.6", "46:33.6", "46:33.7", "46:33.7", "46:33.7", "46:33.8", "46:33.8", "46:33.8", "46:33.9", "46:33.9", "46:33.9", "46:34.0", "46:34.0", "46:34.0", "46:34.1", "46:34.1", "46:34.1", "46:34.2", "46:34.2", "46:34.2", "46:34.3", "46:34.3", "46:34.3", "46:34.4", "46:34.4", "46:34.4", "46:34.5", "46:34.5", "46:34.5", "46:34.6", "46:34.6", "46:34.6", "46:34.7", "46:34.7", "46:34.7", "46:34.8", "46:34.8", "46:34.8", "46:34.9", "46:34.9", "46:34.9", "46:35.0", "46:35.0", "46:35.0", "46:35.1", "46:35.1", "46:35.1", "46:35.2", "46:35.2", "46:35.2", "46:35.3", "46:35.3", "46:35.3", "46:35.4", "46:35.4", "46:35.4", "46:35.5", "46:35.5", "46:35.5", "46:35.6", "46:35.6", "46:35.6", "46:35.7", "46:35.7", "46:35.7", "46:35.8", "46:35.8", "46:35.8", "46:35.9", "46:35.9", "46:35.9", "46:36.0", "46:36.0", "46:36.0", "46:36.1", "46:36.1", "46:36.1", "46:36.2", "46:36.2", "46:36.2", "46:36.3", "46:36.3", "46:36.3", "46:36.4", "46:36.4", "46:36.4", "46:36.5", "46:36.5", "46:36.5", "46:36.6", "46:36.6", "46:36.6", "46:36.7", "46:36.7", "46:36.7", "46:36.8", "46:36.8", "46:36.8", "46:36.9", "46:36.9", "46:36.9", "46:37.0", "46:37.0", "46:37.0", "46:37.1", "46:37.1", "46:37.1", "46:37.2", "46:37.2", "46:37.2", "46:37.3", "46:37.3", "46:37.3", "46:37.4", "46:37.4", "46:37.4", "46:37.5", "46:37.5", "46:37.5", "46:37.6", "46:37.6", "46:37.6", "46:37.7", "46:37.7", "46:37.7", "46:37.8", "46:37.8", "46:37.8", "46:37.9", "46:37.9", "46:37.9", "46:38.0", "46:38.0", "46:38.0", "46:38.1", "46:38.1", "46:38.1", "46:38.2", "46:38.2", "46:38.2", "46:38.3", "46:38.3", "46:38.3", "46:38.4", "46:38.4", "46:38.4", "46:38.5", "46:38.5", "46:38.5", "46:38.6", "46:38.6", "46:38.6", "46:38.7", "46:38.7", "46:38.7", "46:38.8", "46:38.8", "46:38.8", "46:38.9", "46:38.9", "46:38.9", "46:39.0", "46:39.0", "46:39.0", "46:39.1", "46:39.1", "46:39.1", "46:39.2", "46:39.2", "46:39.2", "46:39.3", "46:39.3", "46:39.3", "46:39.4", "46:39.4", "46:39.4", "46:39.5", "46:39.5", "46:39.5", "46:39.6", "46:39.6", "46:39.6", "46:39.7", "46:39.7", "46:39.7", "46:39.8", "46:39.8", "46:39.8", "46:39.9", "46:39.9", "46:39.9", "46:40.0", "46:40.0", "46:40.0", "46:40.1", "46:40.1", "46:40.1", "46:40.2", "46:40.2", "46:40.2", "46:40.3", "46:40.3", "46:40.3", "46:40.4", "46:40.4", "46:40.4", "46:40.5", "46:40.5", "46:40.5", "46:40.6", "46:40.6", "46:40.6", "46:40.7", "46:40.7", "46:40.7", "46:40.8", "46:40.8", "46:40.8", "46:40.9", "46:40.9", "46:40.9", "46:41.0", "46:41.0", "46:41.0", "46:41.1", "46:41.1", "46:41.1", "46:41.2", "46:41.2", "46:41.2", "46:41.3", "46:41.3", "46:41.3", "46:41.4", "46:41.4", "46:41.4", "46:41.5", "46:41.5", "46:41.5", "46:41.6", "46:41.6", "46:41.6", "46:41.7", "46:41.7", "46:41.7", "46:41.8", "46:41.8", "46:41.8", "46:41.9", "46:41.9", "46:41.9", "46:42.0", "46:42.0", "46:42.0", "46:42.1", "46:42.1", "46:42.1", "46:42.2", "46:42.2", "46:42.2", "46:42.3", "46:42.3", "46:42.3", "46:42.4", "46:42.4", "46:42.4", "46:42.5", "46:42.5", "46:42.5", "46:42.6", "46:42.6", "46:42.6", "46:42.7", "46:42.7", "46:42.7", "46:42.8", "46:42.8", "46:42.8", "46:42.9", "46:42.9", "46:42.9", "46:43.0", "46:43.0", "46:43.0", "46:43.1", "46:43.1", "46:43.1", "46:43.2", "46:43.2", "46:43.2", "46:43.3", "46:43.3", "46:43.3", "46:43.4", "46:43.4", "46:43.4", "46:43.5", "46:43.5", "46:43.5", "46:43.6", "46:43.6", "46:43.6", "46:43.7", "46:43.7", "46:43.7", "46:43.8", "46:43.8", "46:43.8", "46:43.9", "46:43.9", "46:43.9", "46:44.0", "46:44.0", "46:44.0", "46:44.1", "46:44.1", "46:44.1", "46:44.2", "46:44.2", "46:44.2", "46:44.3", "46:44.3", "46:44.3", "46:44.4", "46:44.4", "46:44.4", "46:44.5", "46:44.5", "46:44.5", "46:44.6", "46:44.6", "46:44.6", "46:44.7", "46:44.7", "46:44.7", "46:44.8", "46:44.8", "46:44.8", "46:44.9", "46:44.9", "46:44.9", "46:45.0", "46:45.0", "46:45.0", "46:45.1", "46:45.1", "46:45.1", "46:45.2", "46:45.2", "46:45.2", "46:45.3", "46:45.3", "46:45.3", "46:45.4", "46:45.4", "46:45.4", "46:45.5", "46:45.5", "46:45.5", "46:45.6", "46:45.6", "46:45.6", "46:45.7", "46:45.7", "46:45.7", "46:45.8", "46:45.8", "46:45.8", "46:45.9", "46:45.9", "46:45.9", "46:46.0", "46:46.0", "46:46.0", "46:46.1", "46:46.1", "46:46.1", "46:46.2", "46:46.2", "46:46.2", "46:46.3", "46:46.3", "46:46.3", "46:46.4", "46:46.4", "46:46.4", "46:46.5", "46:46.5", "46:46.5", "46:46.6", "46:46.6", "46:46.6", "46:46.7", "46:46.7", "46:46.7", "46:46.8", "46:46.8", "46:46.8", "46:46.9", "46:46.9", "46:46.9", "46:47.0", "46:47.0", "46:47.0", "46:47.1", "46:47.1", "46:47.1", "46:47.2", "46:47.2", "46:47.2", "46:47.3", "46:47.3", "46:47.3", "46:47.4", "46:47.4", "46:47.4", "46:47.5", "46:47.5", "46:47.5", "46:47.6", "46:47.6", "46:47.6", "46:47.7", "46:47.7", "46:47.7", "46:47.8", "46:47.8", "46:47.8", "46:47.9", "46:47.9", "46:47.9", "46:48.0", "46:48.0", "46:48.0", "46:48.1", "46:48.1", "46:48.1", "46:48.2", "46:48.2", "46:48.2", "46:48.3", "46:48.3", "46:48.3", "46:48.4", "46:48.4", "46:48.4", "46:48.5", "46:48.5", "46:48.5", "46:48.6", "46:48.6", "46:48.6", "46:48.7", "46:48.7", "46:48.7", "46:48.8", "46:48.8", "46:48.8", "46:48.9", "46:48.9", "46:48.9", "46:49.0", "46:49.0", "46:49.0", "46:49.1", "46:49.1", "46:49.1", "46:49.2", "46:49.2", "46:49.2", "46:49.3", "46:49.3", "46:49.3", "46:49.4", "46:49.4", "46:49.4", "46:49.5", "46:49.5", "46:49.5", "46:49.6", "46:49.6", "46:49.6", "46:49.7", "46:49.7", "46:49.7", "46:49.8", "46:49.8", "46:49.8", "46:49.9", "46:49.9", "46:49.9", "46:50.0", "46:50.0", "46:50.0", "46:50.1", "46:50.1", "46:50.1", "46:50.2", "46:50.2", "46:50.2", "46:50.3", "46:50.3", "46:50.3", "46:50.4", "46:50.4", "46:50.4", "46:50.5", "46:50.5", "46:50.5", "46:50.6", "46:50.6", 
